vi "Invalidate stdin queue.vi"(1 "connection in":refnum<class "Low Level Connection.lvclass">) -> (0 "connection out":refnum<class "Low Level Connection.lvclass">)   [LabVIEW 2020, in "NI_SFTP.lvlib" / "Low Level Connection.lvclass"]
uses:
  <vilib>/net/SFTP/Low Level Connection/Low Level Connection.lvclass
  <vilib>/net/SFTP/Low Level Connection/Low Level Connection.lvclass/Low Level Connection.ctl
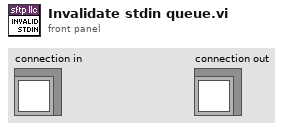
[diagram p1: front panel]
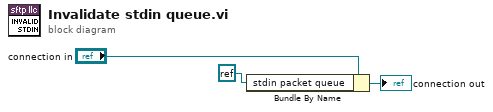
[diagram p0: block diagram]
diagram:
  n1 = Bundle By Name(cluster="connection in", "stdin packet queue"=refnum<k0> refnum) -> (→"connection out":refnum<class "Low Level Connection.lvclass">)
